vi "niTuner Get Temperature with Refresh Interval.vi"(6 "refresh interval":dbl=60.0 format="%.2f", 8 "error in":errorcluster, 9 "correction units":T1(ring)=enum."dBm", 10 "temperature scale":enum16{"Celsius", "Fahrenheit"}(ring), 11 "taskID in":i32=1 format="%.0x") -> (0 "error out":errorcluster {"code" format="%.0x"}, 1 "temperature":dbl format="%.2f", 2 "correction factor":dbl format="%.2p", 3 "taskID out":i32=1 format="%.0x")   [LabVIEW 2011]
doc: "This VI returns the PXI-5600 downconverter temperature at selected intervals and a factor for correcting the temperature response of the PXI-5600 downconverter."
uses:
  nipxi5600u.dll
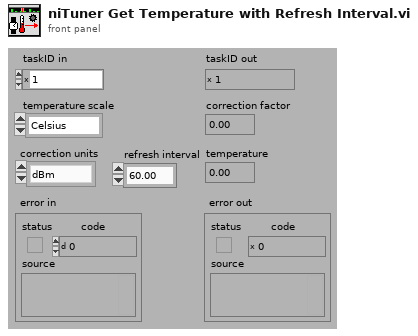
[diagram p1: front panel]
types:
  T1 = enum16{"V", "V^2", "W", "dBm", "dBW", "dBV", "dBmV", "dBuV"}
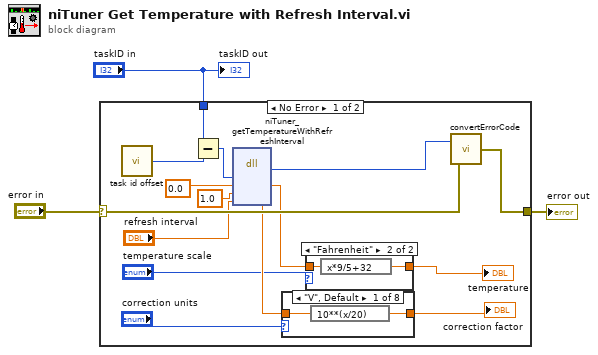
[diagram p0: block diagram]
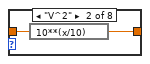
[diagram p3: hidden frame]
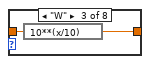
[diagram p4: hidden frame]
diagram:
  n1 = case shown="No Error" "error in" {
    selector: "error in" -> [w17 w33]
    tunnel: [w16 w33] -> w2
    tunnel: "taskID in" -> [w15 _]
    frame No Error {
      n2 = call <instrlib>:"task id offset.vi"() -> ("taskID offset"=w14:i32)
      n3 = Subtract(x=w15, y=w14) -> (x-y=w13:i32)
      n4 = dll-call lib="nipxi5600u.dll" fn="niTuner_getTemperatureWithRefreshInterval"("taskID"=w13, "temperature"=0.0 ("taskID"), "tempCorrectionFactor"=1.0, "refreshInterval"="refresh interval") -> (w18:i32, "temperature"=w5:dbl, "tempCorrectionFactor"=w10:dbl)  [unwired: 5 in, 2 out]
      n5 = case shown="\"V\", Default" "correction units" {
        tunnel: w10 -> [w23 w25 w27 w28 w29 w30 w31 w32]
        tunnel: [w22 w24 w26 w28 w29 w30 w31 w32] -> w8
        frame "V", Default {
          n6 = expression code="10**(x/20)"(w23) -> (w22:dbl)
        }
        frame "V^2" {
          n7 = expression code="10**(x/10)"(w25) -> (w24:dbl)
        }
        frame "W" {
          n8 = expression code="10**(x/10)"(w27) -> (w26:dbl)
        }
        frame "dBm" {
        }
        frame "dBW" {
        }
        frame "dBV" {
        }
        frame "dBmV" {
        }
        frame "dBuV" {
        }
      }
      "correction factor" <- w8
      n9 = case shown="\"Fahrenheit\"" "temperature scale" {
        tunnel: w5 -> [w19 w21]
        tunnel: [w19 w20] -> w6
        frame "Celsius", Default {
        }
        frame "Fahrenheit" {
          n10 = expression code="x*9/5+32"(w21) -> (w20:dbl)
        }
      }
      "temperature" <- w6
      n11 = call <instrlib>:"convertErrorCode.vi"("error in"=w17, "error code"=w18) -> ("error out"=w16:errorcluster)
    }
    frame Error {
    }
  }
  "error out" <- w2
  "taskID out" <- "taskID in"
